vi "Get Field.vi"(8 "error in (no error)":errorcluster, 11 "Instrument.1820 in":refnum<class "Instrument.Oxford1820.lvclass">) -> (0 "error out":errorcluster, 2 "Field (T)":dbl, 3 "Instrument.1820 in":refnum<class "Instrument.Oxford1820.lvclass">)   [LabVIEW 2019, in "Instrument.Oxford1820.lvclass"]
uses:
  Instrument.Oxford1820.lvclass
  C:/Program Files (x86)/National Instruments/LabVIEW 2019/user.lib/LevyLab/Instrument Framework/SMOs/Instrument/Instrument.lvclass
  Typedefs/Instrument.Oxford1820.Commands-enum.ctl
  <userlib>/LevyLab/Instrument Framework/SMOs/Instrument/Instrument.lvclass/Instrument.ctl
  d7882cba-efe1-455e-8983-23068af2cc76.vi
  d7882cba-efe1-455e-8983-23068af2cc76.vi/03a7f0ec-4708-473a-b828-f0ad2cf037a8.vi
  d7882cba-efe1-455e-8983-23068af2cc76.vi/03a7f0ec-4708-473a-b828-f0ad2cf037a8.vi/7d1ffce0-0dca-4f8e-992e-b2e0c96cb3da.vi
  <userlib>/LevyLab/Instrument Framework/SMOs/Instrument/API/Send and Receive.vi
  d7882cba-efe1-455e-8983-23068af2cc76.vi/03a7f0ec-4708-473a-b828-f0ad2cf037a8.vi/85bed98a-4ba7-433f-94d5-52ca6750317c.vi
  <userlib>/LevyLab/Instrument Framework/SMOs/Instrument/Private/Get Client Type.vi
  d7882cba-efe1-455e-8983-23068af2cc76.vi/03a7f0ec-4708-473a-b828-f0ad2cf037a8.vi/7d1ffce0-0dca-4f8e-992e-b2e0c96cb3da.vi/e6e32ba4-1727-462e-b29b-ab4a451f099a.vi
  d7882cba-efe1-455e-8983-23068af2cc76.vi/03a7f0ec-4708-473a-b828-f0ad2cf037a8.vi/7d1ffce0-0dca-4f8e-992e-b2e0c96cb3da.vi/b8b5c2db-f021-4ef8-8420-7280ce2c0ef1.vi
  d7882cba-efe1-455e-8983-23068af2cc76.vi/03a7f0ec-4708-473a-b828-f0ad2cf037a8.vi/85bed98a-4ba7-433f-94d5-52ca6750317c.vi/ca434fa4-036c-4187-8500-86e1d38f8630.vi
  d7882cba-efe1-455e-8983-23068af2cc76.vi/03a7f0ec-4708-473a-b828-f0ad2cf037a8.vi/85bed98a-4ba7-433f-94d5-52ca6750317c.vi/d2b4f1e2-0fa8-4062-bcf5-cc73930e8b7c.vi
  d7882cba-efe1-455e-8983-23068af2cc76.vi/03a7f0ec-4708-473a-b828-f0ad2cf037a8.vi/85bed98a-4ba7-433f-94d5-52ca6750317c.vi/ca434fa4-036c-4187-8500-86e1d38f8630.vi/325892be-d2eb-4425-8653-9ca0c24cbc60.vi
  d7882cba-efe1-455e-8983-23068af2cc76.vi/03a7f0ec-4708-473a-b828-f0ad2cf037a8.vi/85bed98a-4ba7-433f-94d5-52ca6750317c.vi/ca434fa4-036c-4187-8500-86e1d38f8630.vi/6a4e955e-52fc-489f-b28e-4936e5d138b2.vi
  <userlib>/LevyLab/Instrument Framework/SMOs/Instrument/Private/Get RC Connection Status.vi
  <userlib>/LevyLab/Instrument Framework/SMOs/Instrument/API/Enum to String.vi
  <userlib>/LevyLab/Instrument Framework/SMOs/RemoteControl/API/Send and Receive.vi
  <vilib>/Utility/Data Type/Get Type Information.vi
  <vilib>/JDP Science/JSONtext/JSON text to Variant.vi
  <userlib>/LevyLab/Instrument Framework/SMOs/Instrument/API/Instrument.GetPublicEvents.vi
  <vilib>/JDP Science/JSONtext/Variant to JSON Text.vi
  <vilib>/National Instruments/GUID Generator/Guid Generator.vi
  <userlib>/LevyLab/Instrument Framework/SMOs/Instrument/API/Instrument.MessageToProcess.vi
  <userlib>/LevyLab/Instrument Framework/SMOs/Instrument/Private/Instrument.MessageFromProcess.EventStructure.vi
  <vilib>/JDP Science/JSONtext/LVClass Serializer/JSONtext LVClass Serializer.lvclass
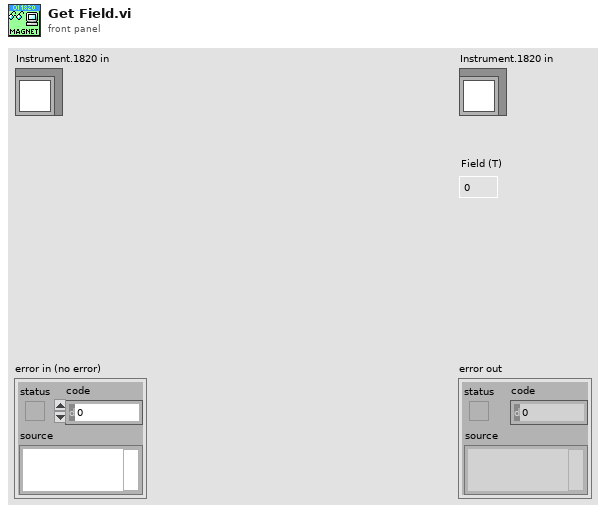
[diagram p1: front panel]
types:
  T1 = typedef "Instrument.Oxford1820.lvclass/Instrument.Oxford1820.Commands-enum.ctl" = enum16{"setAction", "setTarget", "setSwitchHeat", "setLambda", "setFillMode", "setNeedleValve", "setMagnetField", "getStatus", "getTarget", "getSwitchHeat", "getPSUField", "setSequenceStatus", "getMagnetField"}
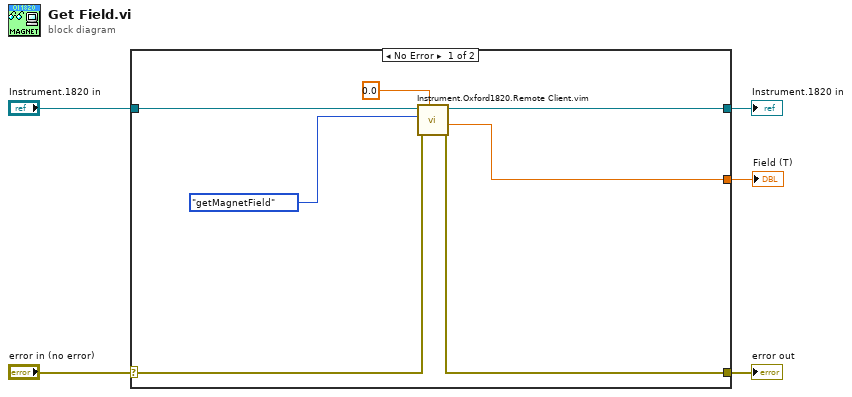
[diagram p0: block diagram]
diagram:
  n1 = case shown="No Error" "error in (no error)" {
    selector: "error in (no error)" -> [w11 w14]
    tunnel: [w6 w14] -> w4
    tunnel: "Instrument.1820 in" -> [w10 w13]
    tunnel: [w7 _] -> w2
    tunnel: [w9 w13] -> w1
    frame No Error {
      n2 = call "Instrument.Oxford1820.Remote Client.vim"("Data Out type"=0.0, "error in (no error)"=w11, "Commands"=Instrument.Oxford1820.Commands-enum."getMagnetField", "Instrument.1820 in"=w10) -> ("error out"=w6:errorcluster, "Data out"=w7:dbl, "Instrument.1820 out"=w9:refnum<class "Instrument.Oxford1820.lvclass">)  [unwired: 5 in]
    }
    frame Error {
    }
  }
  "error out" <- w4
  "Instrument.1820 in" <- w1
  "Field (T)" <- w2
